vi "VerifyClusterWithArrayVariant.vi"(8 "Generated Cluster":cluster{"Array Out":variant[]}, 9 "Cluster In":cluster{"Array In":variant[]}, 10 "String To Append":string, 11 "Base":dbl format="%.2f") -> (3 "All Values Are Equal?":bool)   [LabVIEW 2013]
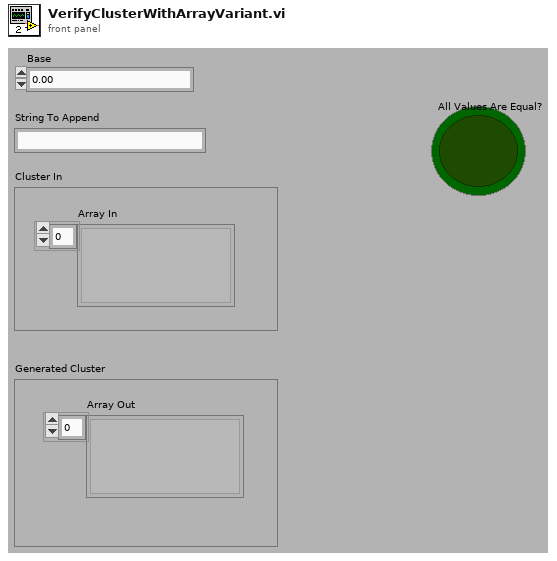
[diagram p1: front panel]
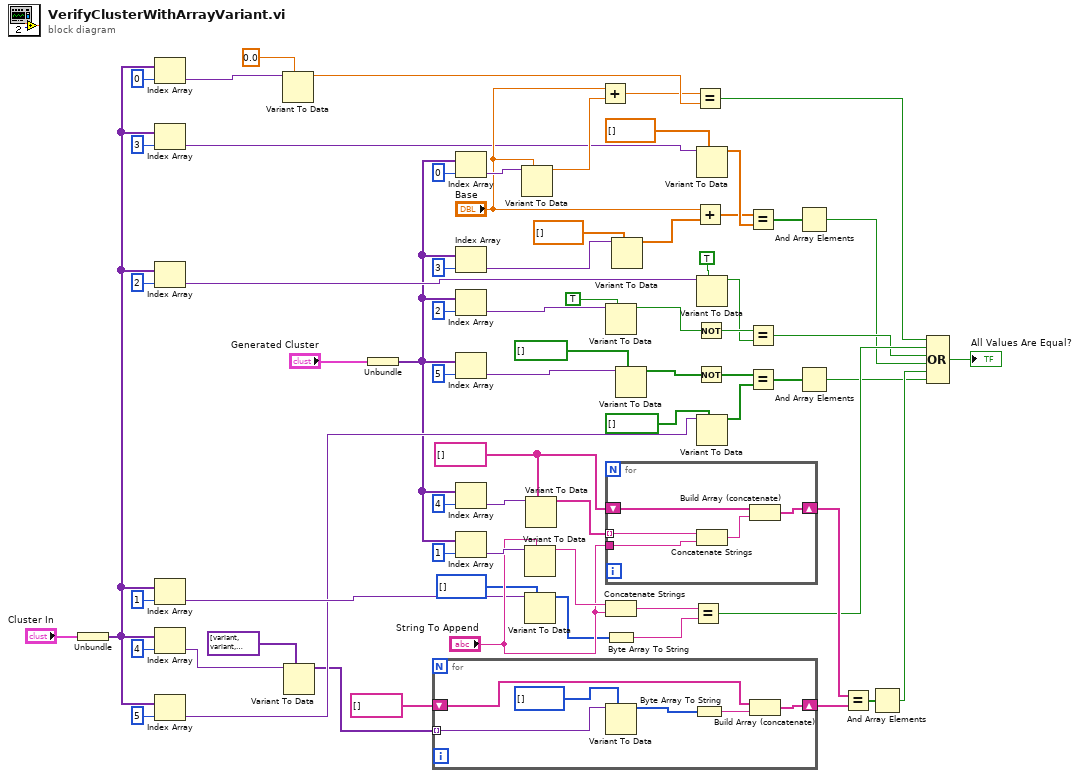
[diagram p0: block diagram]
diagram:
  w52 = string[] []
  n1 = Unbundle("Cluster In") -> ("Array In"=w2:variant[])
  n2 = Index Array(array=w2, index=0) -> (element=w42:variant)
  n3 = Index Array(array=w2, index=3) -> (element=w31:variant)
  n4 = Index Array(array=w2, index=2) -> (element=w35:variant)
  n5 = Index Array(array=w2, index=1) -> (element=w37:variant)
  n6 = Index Array(array=w2, index=4) -> (element=w27:variant)
  n7 = Index Array(array=w2, index=5) -> (element=w24:variant)
  n8 = Variant To Data(type=0.0 ("Base"), Variant=w42) -> (data=w40:dbl)  [unwired: 1 in, 1 out]
  n9 = Variant To Data(type=variant[] [variant, variant, variant, variant, variant, variant] ("Generated Array"), Variant=w27) -> (data=w6:variant[])  [unwired: 1 in, 1 out]
  n10 = Unbundle("Generated Cluster") -> ("Array Out"=w3:variant[])
  n11 = for {
    tunnel: w6 -> [w77] mode=indexing
    shift-right: [w74] -> w5
    shift-left: string[] [] -> [w75]
    n12 = Variant To Data(type=u8[] [] ("x+y"), Variant=w77) -> (data=w73:u8[])  [unwired: 1 in, 1 out]
    n13 = Byte Array To String(unsigned byte array=w73) -> (string=w72:string)
    n14 = Build Array (concatenate)(w75, w72) -> (w74:string[])
  }
  n15 = Index Array(array=w3, index=0) -> (element=w70:variant)
  n16 = Index Array(array=w3, index=3) -> (element=w60:variant)
  n17 = Index Array(array=w3, index=2) -> (element=w64:variant)
  n18 = Index Array(array=w3, index=5) -> (element=w50:variant)
  n19 = Index Array(array=w3, index=4) -> (element=w54:variant)
  n20 = Index Array(array=w3, index=1) -> (element=w67:variant)
  n21 = Variant To Data(type="Base", Variant=w70) -> (data=w69:dbl)  [unwired: 1 in, 1 out]
  n22 = Variant To Data(type="String To Append", Variant=w67) -> (data=w66:string)  [unwired: 1 in, 1 out]
  n23 = Variant To Data(type=u8[] [] ("x+y"), Variant=w37) -> (data=w36:u8[])  [unwired: 1 in, 1 out]
  n24 = Variant To Data(type=w52, Variant=w54) -> (data=w53:string[])  [unwired: 1 in, 1 out]
  n25 = Add(x="Base", y=w69) -> (x+y=w39:dbl)
  n26 = Variant To Data(type=TRUE, Variant=w64) -> (data=w62:bool)  [unwired: 1 in, 1 out]
  n27 = for {
    tunnel: w53 -> [w82] mode=indexing
    shift-right: [w78] -> w26
    shift-left: w52 -> [w79]
    tunnel: "String To Append" -> [w81]
    n28 = Concatenate Strings(w82, w81) -> (w80:string)
    n29 = Build Array (concatenate)(w79, w80) -> (w78:string[])
  }
  n30 = Concatenate Strings(w66, "String To Append") -> (w38:string)
  n31 = Byte Array To String(unsigned byte array=w36) -> (string=w9:string)
  n32 = Variant To Data(type=dbl[] [], Variant=w60) -> (data=w58:dbl[])  [unwired: 1 in, 1 out]
  n33 = Variant To Data(type=bool[] [], Variant=w50) -> (data=w48:bool[])  [unwired: 1 in, 1 out]
  n34 = Equal?(x=w38, y=w9) -> (x = y?=w16:bool)
  n35 = Equal?(x=w39, y=w40) -> (x = y?=w17:bool)
  n36 = Add(x="Base", y=w58) -> (x+y=w28:dbl[])
  n37 = Not(x=w62) -> (.not. x?=w33:bool)
  n38 = Not(x=w48) -> (.not. x?=w21:bool[])
  n39 = Variant To Data(type=dbl[] [] ("x+y"), Variant=w31) -> (data=w29:dbl[])  [unwired: 1 in, 1 out]
  n40 = Variant To Data(type=TRUE, Variant=w35) -> (data=w32:bool)  [unwired: 1 in, 1 out]
  n41 = Variant To Data(type=bool[] [], Variant=w24) -> (data=w22:bool[])  [unwired: 1 in, 1 out]
  n42 = Equal?(x=w28, y=w29) -> (x = y?=w20:bool[])
  n43 = Equal?(x=w33, y=w32) -> (x = y?=w15:bool)
  n44 = Equal?(x=w21, y=w22) -> (x = y?=w18:bool[])
  n45 = And Array Elements(Boolean array=w20) -> (logical AND=w14:bool)
  n46 = And Array Elements(Boolean array=w18) -> (logical AND=w12:bool)
  n47 = Equal?(x=w26, y=w5) -> (x = y?=w19:bool[])
  n48 = And Array Elements(Boolean array=w19) -> (logical AND=w13:bool)
  n49 = Compound Arithmetic op=OR(w17, w16, w15, w14, w13, w12) -> (→"All Values Are Equal?":bool)
